vi "Load People.vi"(3 "errorIN":errorcluster, 5 "Employee array":refnum<vi>[](array[refnum])) -> (0 "error OUT":errorcluster, 2 "Employees":string[](array[string]))   [LabVIEW 2010]
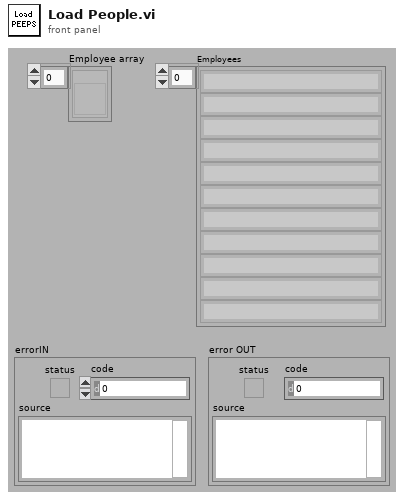
[diagram p1: front panel]
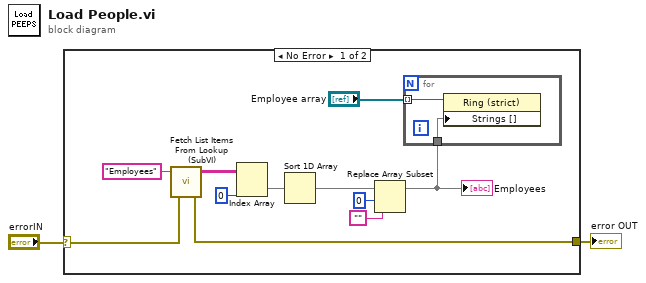
[diagram p0: block diagram]
diagram:
  n1 = case shown="No Error" "errorIN" {
    selector: "errorIN" -> [w9 w16]
    tunnel: [w8 w16] -> w1
    frame No Error {
      n2 = call "Fetch List Items From Lookup (SubVI).vi"("error IN"=w9, "Query"="Employees" ("lookup table name")) -> ("error OUT"=w8:errorcluster, "recordset data"=w13:string[][])  [unwired: 2 out]
      n3 = Index Array(array=w13, index (col)=0 ("disabled index (col)")) -> (element=w10:string[])  [unwired: 1 in]
      n4 = Sort 1D Array(array=w10) -> (sorted array=w4:string[])
      n5 = Replace Array Subset(array=w4, new element="" ("new element/subarray"), index=0) -> (w3:string[])
      "Employees" <- w3
      n6 = for {
        tunnel: "Employee array" -> [w15] mode=indexing
        tunnel: w3 -> [w14]
        n7 = property class="Ring (strict)"(reference=w15, "Strings []"=w14) -> ()  [unwired: 1 in, 2 out]
      }
    }
    frame Error {
    }
  }
  "error OUT" <- w1
